vi "GFG 2012 or 2014 or 2015.vi"   [LabVIEW 2012]
doc: "SciScan 1.2 160622"
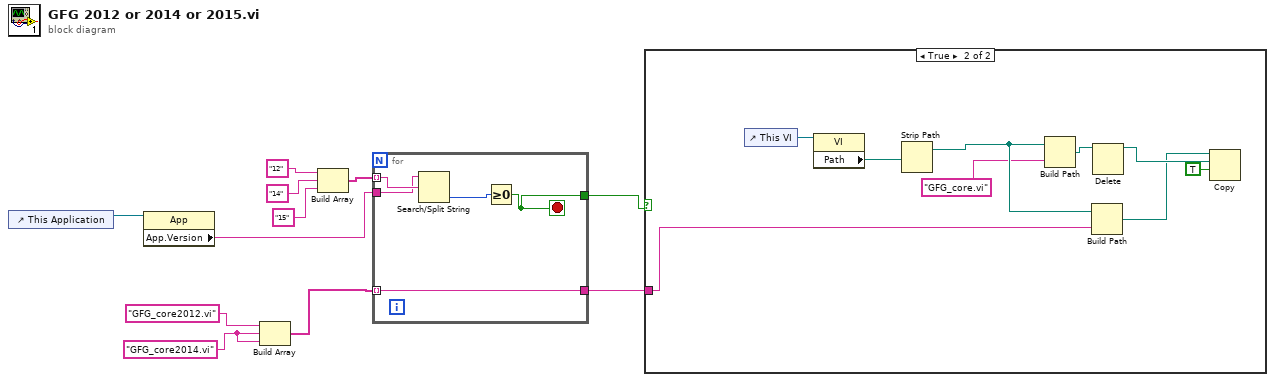
[diagram p0: block diagram]
diagram:
  w1 = "GFG_core2014.vi" ("name or relative path")
  n1 = control-ref of="This Application"() -> (w6:refnum<vi>)
  n2 = property class="App"(reference=w6) -> ("App.Version"=w10:string)  [unwired: 1 in, 2 out]
  n3 = Build Array("GFG_core2012.vi" ("t"), w1, w1) -> (w5:string[])
  n4 = Build Array("12" ("F button name (\"Cancel\")"), "14" ("F button name (\"Cancel\")"), "15" ("element")) -> (w9:string[])
  n5 = for {
    tunnel: w9 -> [w16] mode=indexing
    tunnel: w10 -> [w15]
    tunnel: w5 -> [w13] mode=indexing
    tunnel: [w13] -> w3
    tunnel: [w12] -> w4
    stop <- w12 stop-if-true
    n6 = Search/Split String(string=w15, search string/char (-)=w16) -> (offset of match=w14:i32)  [unwired: 1 in, 2 out]
    n7 = Greater Or Equal To 0?(x=w14) -> (x >= 0?=w12:bool)
  }
  n8 = case shown="True" w4 {
    tunnel: w3 -> [_ w18]
    frame False {
    }
    frame True {
      n9 = control-ref of="This VI"() -> (w25:refnum<vi>)
      n10 = property class="VI"(reference=w25) -> ("Path"=w24:path)  [unwired: 1 in, 2 out]
      n11 = Strip Path(path=w24) -> (stripped path=w21:path)  [unwired: 1 out]
      n12 = Build Path(base path=w21, name or relative path="GFG_core.vi") -> (appended path=w22:path)
      n13 = Build Path(base path=w21, name or relative path=w18) -> (appended path=w17:path)
      n14 = Delete(path (use dialog)=w22) -> (deleted path=w19:path)  [unwired: 4 in, 2 out]
      n15 = Copy(9:TRUE ("overwrite (F)"), 10:w19, 11:w17) -> ()  [unwired: 2 in, 3 out]
    }
  }
